vi "Reroll BaseNodeType Identifiers.vi"(8 "error in":errorcluster, 11 "BaseNodeType in":refnum<k39>) -> (0 "error out":errorcluster, 3 "BaseNodeType out":refnum<k39>)   [LabVIEW 2020, in "Custom Device Serialization.lvlib"]
uses:
  Custom Device Serialization.lvlib
  C:/NetCoreDLL/NationalInstruments.VeriStand.SystemStorage.dll
  NetCoreDLL/NationalInstruments.VeriStand.SystemStorage.dll
  C:/Program Files/dotnet/shared/Microsoft.NETCore.App/10.0.12/System.Private.CoreLib.dll
  Program Files/dotnet/shared/Microsoft.NETCore.App/10.0.12/System.Private.CoreLib.dll
  C:/Program Files/dotnet/shared/Microsoft.NETCore.App/10.0.12/mscorlib.dll
  Program Files/dotnet/shared/Microsoft.NETCore.App/10.0.12/mscorlib.dll
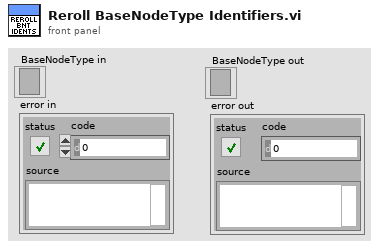
[diagram p1: front panel]
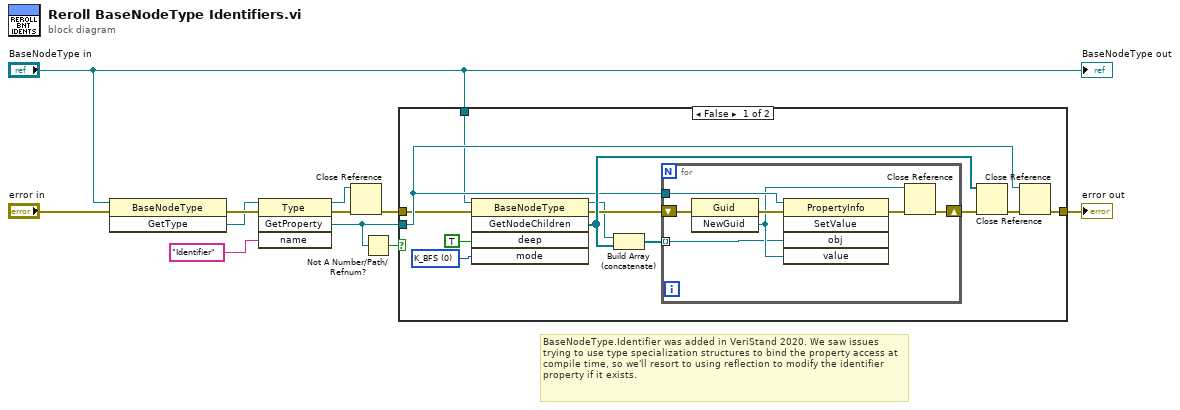
[diagram p0: block diagram]
diagram:
  # "BaseNodeType.Identifier was added in VeriStand 2020. We saw issues trying to use type specialization structures to bind the property access at compile time, so we'll resort to using reflection to modify the identifier property if it exists."
  n1 = invoke class="BaseNodeType" method="GetType"(reference="BaseNodeType in", error in="error in") -> (error out=w10:errorcluster, "GetType"=w9:refnum<k39>)  [unwired: 1 in, 1 out]
  n2 = invoke class="Type" method="GetProperty"(reference=w9, error in=w10, "name"="Identifier") -> (reference out=w6:refnum<k39>, error out=w7:errorcluster, "GetProperty"=w1:refnum<k39>)  [unwired: 1 in, 1 out]
  n3 = Close Reference(reference=w6, error in (no error)=w7) -> (error out=w4:errorcluster)
  n4 = Not A Number/Path/Refnum?(number/path/refnum=w1) -> (NaN/Path/Refnum?=w2:bool)
  n5 = case shown="False" w2 {
    tunnel: [w12 w31] -> w11
    tunnel: w1 -> [w19 _]
    tunnel: w4 -> [w18 w31]
    tunnel: "BaseNodeType in" -> [w15 _]
    frame False {
      w21 = 0 items=["K_BFS", "K_DFS", "K_CHILDONLY", "K_UP"] ("mode")
      n6 = invoke class="BaseNodeType" method="GetNodeChildren"(reference=w15, error in=w18, "deep"=TRUE, "mode"=w21) -> (reference out=w16:refnum<k39>, error out=w17:errorcluster, "GetNodeChildren"=w23:refnum<k39>[])  [unwired: 1 in, 2 out]
      n7 = Build Array (concatenate)(w16, w23) -> (w20:refnum<k39>[])
      n8 = for {
        tunnel: w20 -> [w24] mode=indexing
        shift-right: [w30] -> w14
        shift-left: w17 -> [w29]
        tunnel: w19 -> [w28]
        n9 = invoke class="Guid" method="NewGuid"(error in=w29) -> (error out=w27:errorcluster, "NewGuid"=w26:refnum<k39>)  [unwired: 2 in, 1 out]
        n10 = invoke class="PropertyInfo" method="SetValue"(reference=w28, error in=w27, "obj"=w24, "value"=w26) -> (error out=w25:errorcluster)  [unwired: 1 in, 4 out]
        n11 = Close Reference(reference=w26, error in (no error)=w25) -> (error out=w30:errorcluster)
      }
      n12 = Close Reference(reference=w23, error in (no error)=w14) -> (error out=w13:errorcluster)
      n13 = Close Reference(reference=w19, error in (no error)=w13) -> (error out=w12:errorcluster)
    }
    frame True {
    }
  }
  "error out" <- w11
  "BaseNodeType out" <- "BaseNodeType in"
